vi "Configure Marker Type (Others).vi"(0 "VISA resource name":refnum<visa-resource-name>, 1 "X-axis Value (0)":dbl, 5 "Active Marker (1: Marker1)":i32(ring)=1 items=["Marker1"=1, "Marker2"=2, "Marker3"=3, "Marker4"=4, "Marker5"=5, "Marker6"=6, "Marker7"=7, "Marker8"=8, "Marker9"=9, "Marker10"=10, "Marker11"=11, "Marker12"=12], 7 "Marker Type (0: Normal)":i32(ring) items=["Normal", "Delta", "Off"], 9 "Reference Marker (1: Marker1)":i32(ring)=1 items=["Marker1"=1, "Marker2"=2, "Marker3"=3, "Marker4"=4, "Marker5"=5, "Marker6"=6, "Marker7"=7, "Marker8"=8, "Marker9"=9, "Marker10"=10, "Marker11"=11, "Marker12"=12], 11 "error in (no error)":errorcluster) -> (4 "VISA resource name out":refnum<visa-resource-name>, 15 "error out":errorcluster)   [LabVIEW 2018, in "Agilent MXA Series.lvlib"]
doc: "Configures the marker type on the spectrum analyzer.\n\n<B>Note:</B>\nYou can use this VI under Channel Power Measurement, Occupied Bandwith, Power Stat CCDF, ACP, Burst Power, Spurious Emissions and Spectrum Emission Mask measurement types."
uses:
  Agilent MXA Series.lvlib
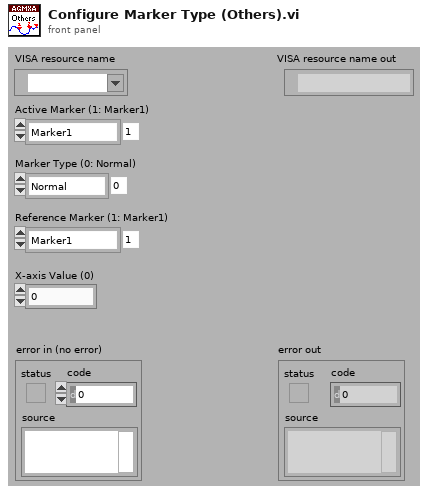
[diagram p1: front panel]
types:
  T1 = typedef "Agilent MXA Series.lvlib/Extended User Data.ctl" = cluster{"Measurement Type":i32, "Agilent MXA/EXA Model":i32}
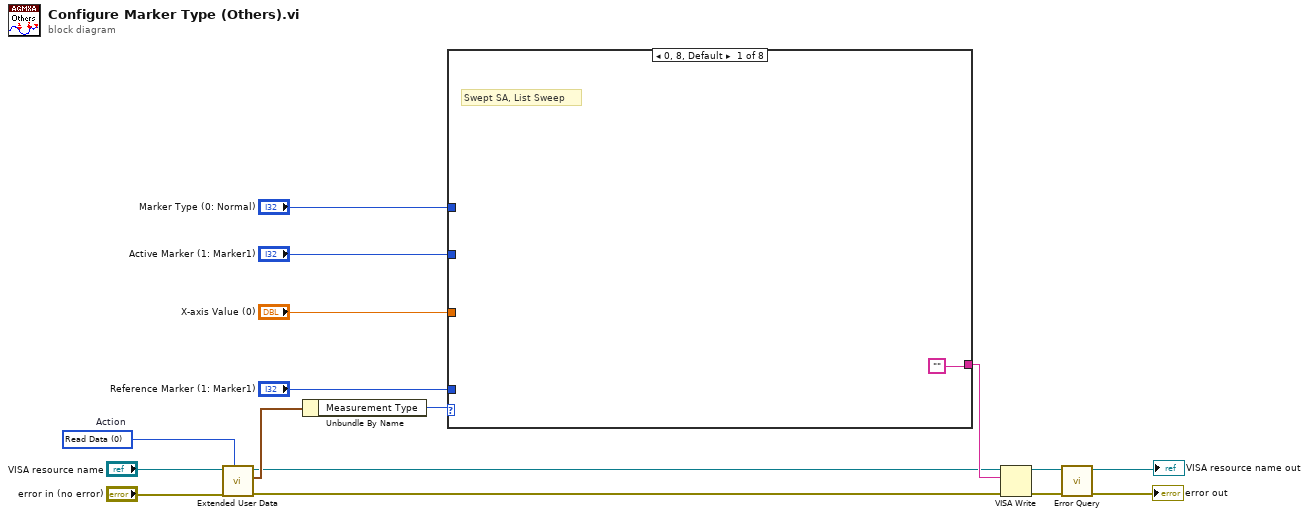
[diagram p0: block diagram]
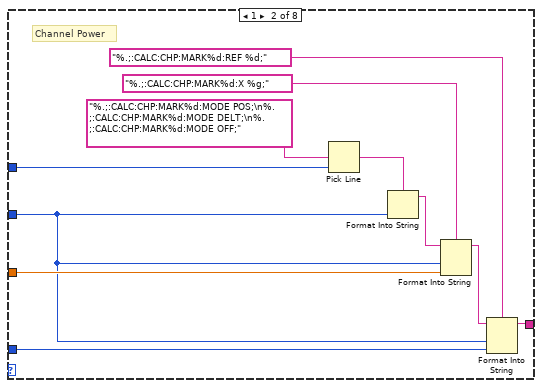
[diagram p2: hidden frame]
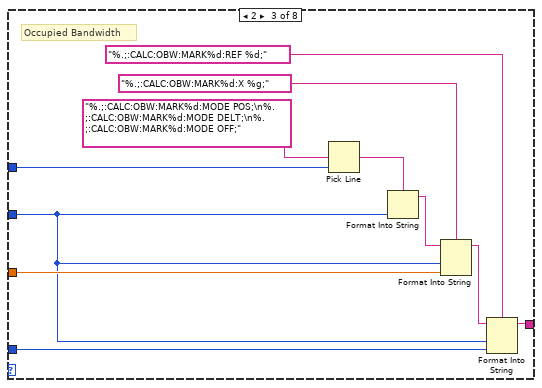
[diagram p3: hidden frame]
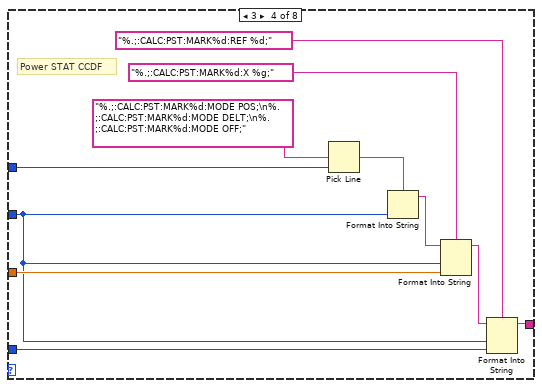
[diagram p4: hidden frame]
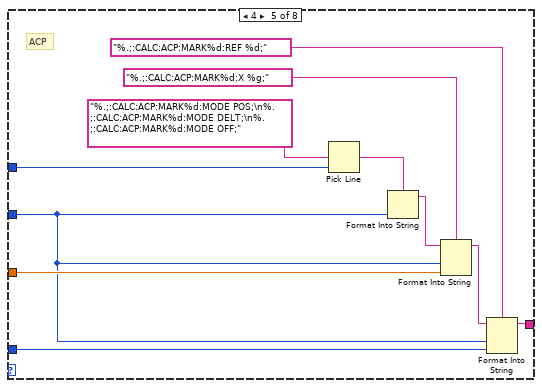
[diagram p5: hidden frame]
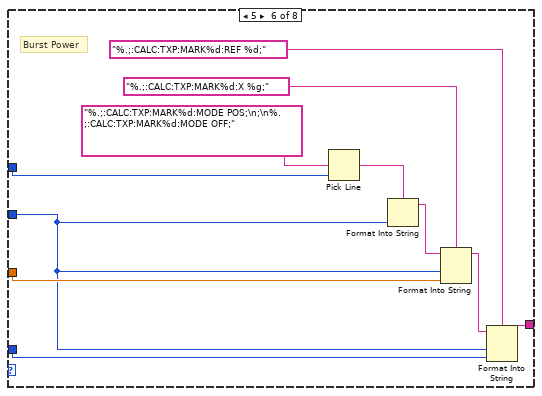
[diagram p6: hidden frame]
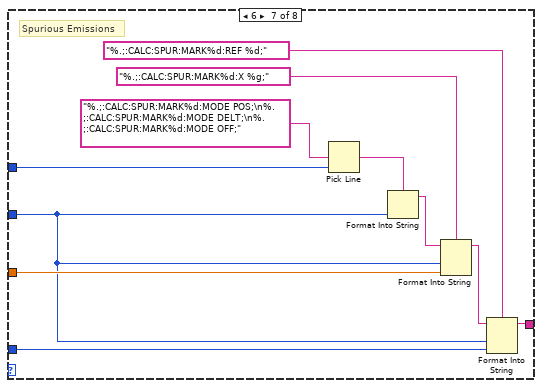
[diagram p7: hidden frame]
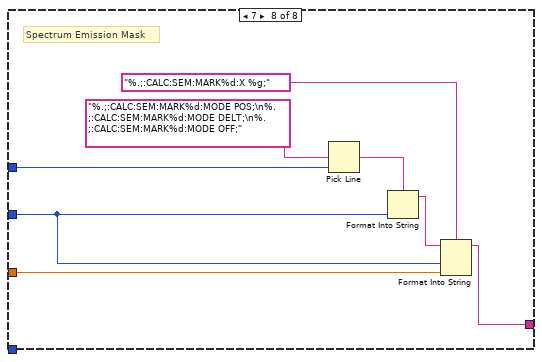
[diagram p8: hidden frame]
diagram:
  w14 = 0 items=["Read Data", "Write Data", "Clear Data", "Clear ALL Data"]  # Action
  n1 = call "Extended User Data.vi"("Action (1:Write Data)"=w14, "Error In (no error)"="error in (no error)", "VISA resource name in"="VISA resource name") -> ("Error Out"=w3:errorcluster, "User Data Out"=w13:T1, "VISA resource name out"=w2:refnum<visa-resource-name>)  [unwired: 6 in]
  n2 = Unbundle By Name(w13) -> ("Measurement Type"=w12:i32)
  n3 = case shown="0, 8, Default" w12 {
    tunnel: "Marker Type (0: Normal)" -> [_ w28 w39 w50 w61 w72 w83 w91]
    tunnel: "Active Marker (1: Marker1)" -> [_ w21 w32 w41 w54 w65 w76 w85]
    tunnel: "X-axis Value (0)" -> [_ w23 w34 w45 w56 w67 w78 w86]
    tunnel: ["" w18 w29 w40 w51 w62 w73 w84] -> w4
    tunnel: "Reference Marker (1: Marker1)" -> [_ w20 w31 w43 w53 w64 w75 _]
    frame 0, 8, Default {
      # "Swept SA, List Sweep"
    }
    frame 1 {
      # "Channel Power"
      n4 = Pick Line(multi-line string="%.;:CALC:CHP:MARK%d:MODE POS;\n%.;:CALC:CHP:MARK%d:MODE DELT;\n%.;:CALC:CHP:MARK%d:MODE OFF;", line index=w28) -> (output string=w26:string)  [unwired: 1 in]
      n5 = Format Into String(format string=w26, w21) -> (resulting string=w24:string)  [unwired: 2 in, 1 out]
      n6 = Format Into String(format string="%.;:CALC:CHP:MARK%d:X %g;", initial string=w24, w21, w23) -> (resulting string=w19:string)  [unwired: 1 in, 1 out]
      n7 = Format Into String(format string="%.;:CALC:CHP:MARK%d:REF %d;", initial string=w19, w21, w20) -> (resulting string=w18:string)  [unwired: 1 in, 1 out]
    }
    frame 2 {
      # "Occupied Bandwidth"
      n8 = Pick Line(multi-line string="%.;:CALC:OBW:MARK%d:MODE POS;\n%.;:CALC:OBW:MARK%d:MODE DELT;\n%.;:CALC:OBW:MARK%d:MODE OFF;", line index=w39) -> (output string=w37:string)  [unwired: 1 in]
      n9 = Format Into String(format string=w37, w32) -> (resulting string=w35:string)  [unwired: 2 in, 1 out]
      n10 = Format Into String(format string="%.;:CALC:OBW:MARK%d:X %g;", initial string=w35, w32, w34) -> (resulting string=w30:string)  [unwired: 1 in, 1 out]
      n11 = Format Into String(format string="%.;:CALC:OBW:MARK%d:REF %d;", initial string=w30, w32, w31) -> (resulting string=w29:string)  [unwired: 1 in, 1 out]
    }
    frame 3 {
      # "Power STAT CCDF"
      n12 = Pick Line(multi-line string="%.;:CALC:PST:MARK%d:MODE POS;\n%.;:CALC:PST:MARK%d:MODE DELT;\n%.;:CALC:PST:MARK%d:MODE OFF;", line index=w50) -> (output string=w48:string)  [unwired: 1 in]
      n13 = Format Into String(format string=w48, w41) -> (resulting string=w46:string)  [unwired: 2 in, 1 out]
      n14 = Format Into String(format string="%.;:CALC:PST:MARK%d:X %g;", initial string=w46, w41, w45) -> (resulting string=w42:string)  [unwired: 1 in, 1 out]
      n15 = Format Into String(format string="%.;:CALC:PST:MARK%d:REF %d;", initial string=w42, w41, w43) -> (resulting string=w40:string)  [unwired: 1 in, 1 out]
    }
    frame 4 {
      # "ACP"
      n16 = Pick Line(multi-line string="%.;:CALC:ACP:MARK%d:MODE POS;\n%.;:CALC:ACP:MARK%d:MODE DELT;\n%.;:CALC:ACP:MARK%d:MODE OFF;", line index=w61) -> (output string=w59:string)  [unwired: 1 in]
      n17 = Format Into String(format string=w59, w54) -> (resulting string=w57:string)  [unwired: 2 in, 1 out]
      n18 = Format Into String(format string="%.;:CALC:ACP:MARK%d:X %g;", initial string=w57, w54, w56) -> (resulting string=w52:string)  [unwired: 1 in, 1 out]
      n19 = Format Into String(format string="%.;:CALC:ACP:MARK%d:REF %d;", initial string=w52, w54, w53) -> (resulting string=w51:string)  [unwired: 1 in, 1 out]
    }
    frame 5 {
      # "Burst Power"
      n20 = Pick Line(multi-line string="%.;:CALC:TXP:MARK%d:MODE POS;\n;\n%.;:CALC:TXP:MARK%d:MODE OFF;", line index=w72) -> (output string=w70:string)  [unwired: 1 in]
      n21 = Format Into String(format string=w70, w65) -> (resulting string=w68:string)  [unwired: 2 in, 1 out]
      n22 = Format Into String(format string="%.;:CALC:TXP:MARK%d:X %g;", initial string=w68, w65, w67) -> (resulting string=w63:string)  [unwired: 1 in, 1 out]
      n23 = Format Into String(format string="%.;:CALC:TXP:MARK%d:REF %d;", initial string=w63, w65, w64) -> (resulting string=w62:string)  [unwired: 1 in, 1 out]
    }
    frame 6 {
      # "Spurious Emissions"
      n24 = Pick Line(multi-line string="%.;:CALC:SPUR:MARK%d:MODE POS;\n%.;:CALC:SPUR:MARK%d:MODE DELT;\n%.;:CALC:SPUR:MARK%d:MODE OFF;", line index=w83) -> (output string=w81:string)  [unwired: 1 in]
      n25 = Format Into String(format string=w81, w76) -> (resulting string=w79:string)  [unwired: 2 in, 1 out]
      n26 = Format Into String(format string="%.;:CALC:SPUR:MARK%d:X %g;", initial string=w79, w76, w78) -> (resulting string=w74:string)  [unwired: 1 in, 1 out]
      n27 = Format Into String(format string="%.;:CALC:SPUR:MARK%d:REF %d;", initial string=w74, w76, w75) -> (resulting string=w73:string)  [unwired: 1 in, 1 out]
    }
    frame 7 {
      # "Spectrum Emission Mask"
      n28 = Pick Line(multi-line string="%.;:CALC:SEM:MARK%d:MODE POS;\n%.;:CALC:SEM:MARK%d:MODE DELT;\n%.;:CALC:SEM:MARK%d:MODE OFF;", line index=w91) -> (output string=w89:string)  [unwired: 1 in]
      n29 = Format Into String(format string=w89, w85) -> (resulting string=w87:string)  [unwired: 2 in, 1 out]
      n30 = Format Into String(format string="%.;:CALC:SEM:MARK%d:X %g;", initial string=w87, w85, w86) -> (resulting string=w84:string)  [unwired: 1 in, 1 out]
    }
  }
  n31 = VISA Write(VISA resource name=w2, write buffer=w4, error in (no error)=w3) -> (VISA resource name out=w8:refnum<visa-resource-name>, error out=w7:errorcluster)  [unwired: 1 out]
  n32 = call "Error Query.vi"("error in (no error)"=w7, "VISA resource name"=w8) -> ("error out"=→"error out":errorcluster, "VISA resource name out"=→"VISA resource name out":refnum<visa-resource-name>)  [unwired: 6 in, 2 out]
